vi "vision_webcam_V6.vi"() -> ()   [LabVIEW 2017]
uses:
  <vilib>/userdefined/High Color/IMAQdx.ctl
  <vilib>/vision/Image Controls.llb/IMAQ Image.ctl
  <vilib>/vision/Avi.llb/IMAQ AVI2 Codec Path.ctl
  Globals/Global - All RT Loop Stop.vi
  <vilib>/vision/driver/NI_Vision_Acquisition_Software.lvlib
panel:
  out "error out":errorcluster
  in  "y":bool
  out "AVI Path":path
  out "concatenated string 2":string
  in  "Boolean":bool
  out "Codec Names":string[](array[string])
  out "Webcam":T1(plugin-control)
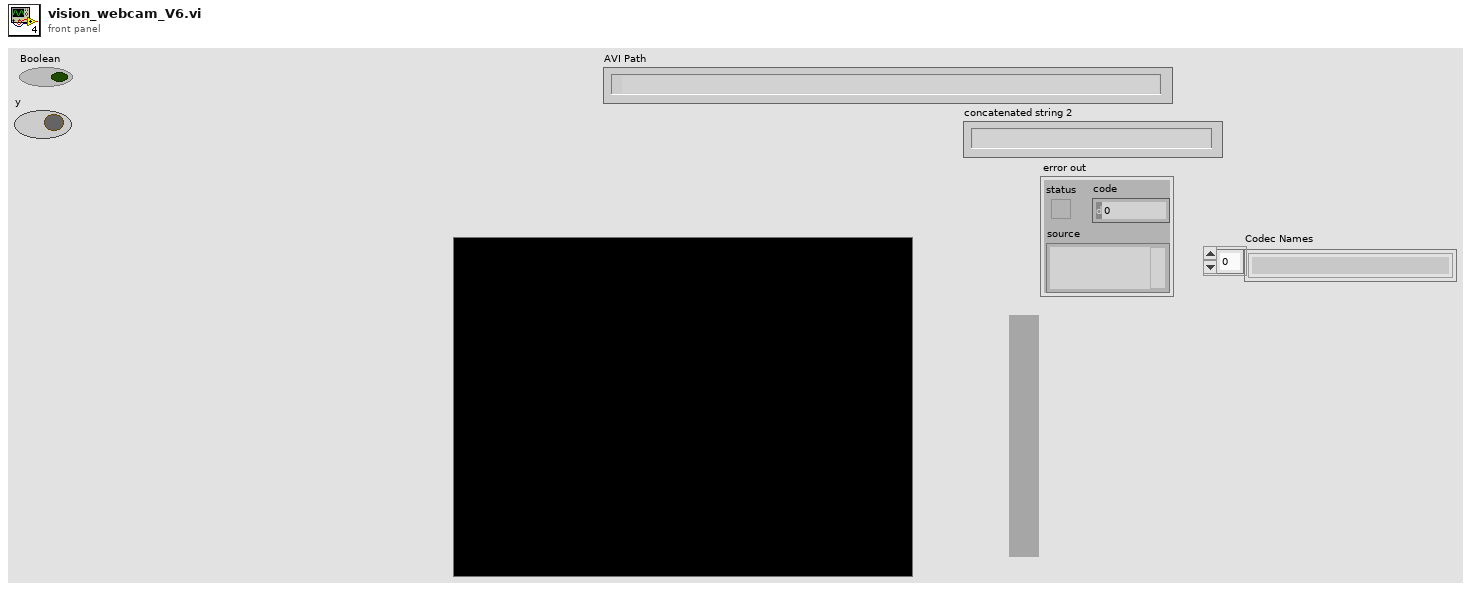
[diagram p1: front panel]
types:
  T1 = typedef "IMAQ Image.ctl" = refnum<image>
  T2 = typedef "IMAQdx.ctl" = refnum<k21>
  T3 = typedef "Image Type" = u32
  T4 = typedef "IMAQ AVI2 Refnum.ctl" = refnum<k20>
  T5 = typedef "IMAQ AVI2 Codec Path.ctl" = u32
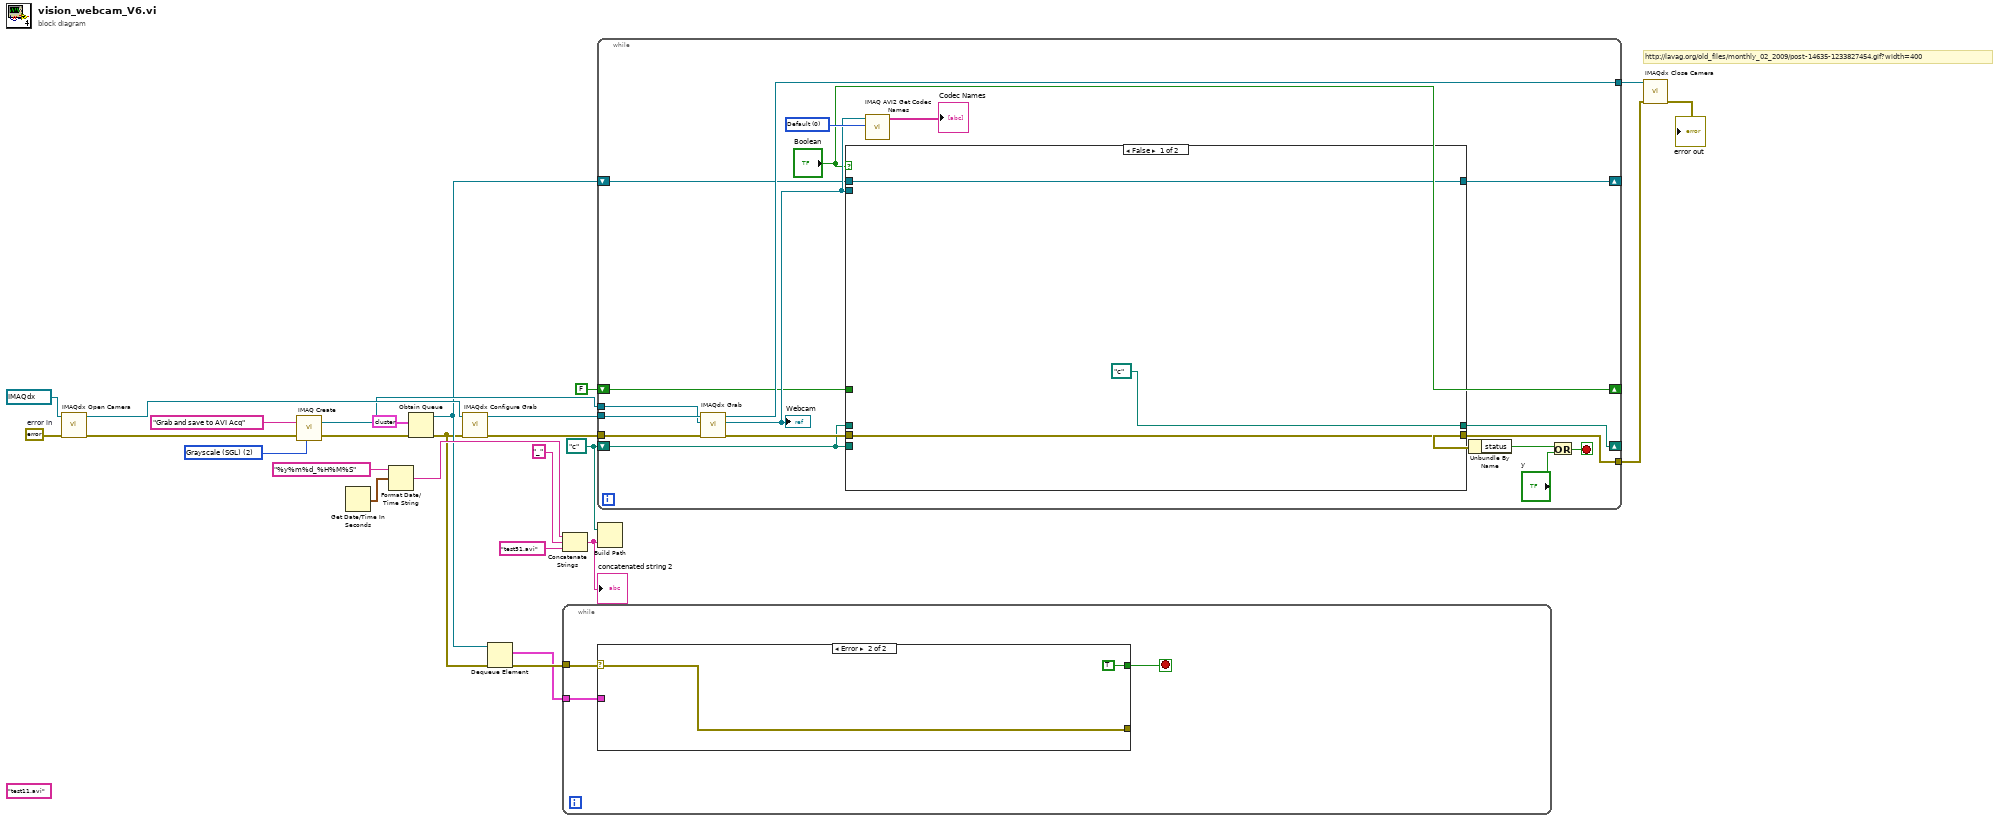
[diagram p0: block diagram]
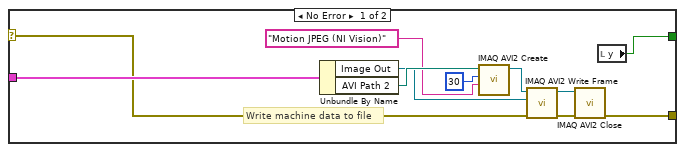
[diagram p2: hidden frame]
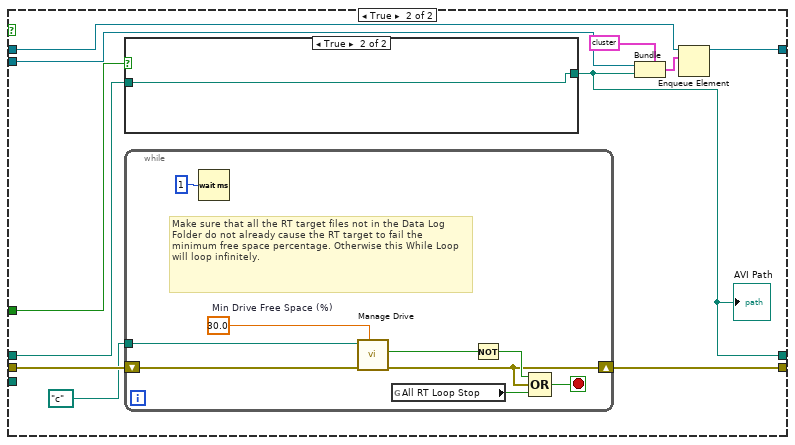
[diagram p3: hidden frame]
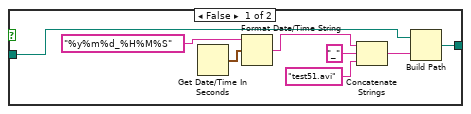
[diagram p4: hidden frame]
diagram:
  (unwired) "test11.avi" ("name or relative path")
  w11 = path "c:/" ("AVI Path")
  w21 = T3 2 items=["Grayscale (U8)", "Grayscale (I16)", "Grayscale (SGL)", "Complex (CSG)", "RGB (U32)", "HSL (U32)", "RGB (U64)", "Grayscale (U16)"] ("Image Type")
  w23 = errorcluster {"status"=FALSE, "code"=0, "source"=""}  # error in
  # "http://lavag.org/old_files/monthly_02_2009/post-14635-1233827454.gif?width=400"
  n1 = call <vilib>:"IMAQdx Open Camera.vi"("error in"=w23, "Session In"=T2 "cam0") -> ("error out"=w20:errorcluster, "Session Out"=w25:T2)  [unwired: 8 in]
  n2 = call "IMAQ Create"("Image Name"="Grab and save to AVI Acq", "Image Type"=w21, "error in (no error)"=w20) -> ("New Image"=w17:T1, "error out"=w4:errorcluster)  [unwired: 2 in]
  n3 = Get Date/Time In Seconds() -> (seconds since 1Jan1904=w15:timestamp)
  n4 = Format Date/Time String(time format string (%c)="%y%m%d_%H%M%S", seconds (now)=w15) -> (date/time string=w14:string)  [unwired: 1 out]
  n5 = Obtain Queue(element data type=cluster{"Image Out":T1, "AVI Path 2":path} {"Image Out"=refnum, "AVI Path 2"=path ""}, error in (no error)=w4) -> (queue out=w5:refnum<queue>, error out=w3:errorcluster)  [unwired: 3 in, 1 out]
  n6 = call <vilib>:"IMAQdx Configure Grab.vi"("error in"=w3, "Session In"=w25) -> ("error out"=w18:errorcluster, "Session Out"=w19:T2)  [unwired: 8 in]
  n7 = Dequeue Element(queue=w5, error in (no error)=w3) -> (element=w6:cluster{"Image Out":T1, "AVI Path 2":path}, error out=w7:errorcluster)  [unwired: 1 in, 2 out]
  n8 = Concatenate Strings(w14, "_" ("string"), "test51.avi" ("name or relative path")) -> (w10:string)
  "concatenated string 2" <- w10
  n9 = while {
    tunnel: w7 -> [w29]
    tunnel: w6 -> [w28]
    stop <- w27 stop-if-true
    n10 = case shown="Error" w29 {
      selector: w29 -> [w34 w42]
      tunnel: [w31 w42] -> _
      tunnel: w28 -> [w40 _]
      tunnel: [w30 TRUE] -> w27
      frame No Error {
        # "Write machine data to file"
        n11 = Unbundle By Name(w40) -> ("Image Out"=w35:T1, "AVI Path 2"=w39:path)
        n12 = call "IMAQ AVI2 Create"("Codec"="Motion JPEG (NI Vision)", "Frames Per Second"=u32 30, "AVI Path"=w39) -> ("AVI Refnum"=w36:T4)  [unwired: 7 in, 1 out]
        n13 = call "IMAQ AVI2 Write Frame"("error in (no error)"=w34, "Image"=w35, "AVI Refnum"=w36) -> ("error out"=w32:errorcluster, "AVI Refnum (duplicate)"=w33:T4)  [unwired: 6 in, 1 out]
        n14 = call "IMAQ AVI2 Close"("error in (no error)"=w32, "AVI Refnum"=w33) -> ("error out"=w31:errorcluster)  [unwired: 9 in]
        n15 = local read "y"() -> (w30:bool)
      }
      frame Error {
      }
    }
  }
  n16 = while {
    tunnel: w18 -> [w60]
    tunnel: w19 -> [w59]
    tunnel: w17 -> [w58]
    tunnel: [w50] -> w2
    tunnel: [w57] -> w26
    shift-right: [w48] -> _
    shift-left: w5 -> [w49]
    shift-right: ["Boolean"] -> _
    shift-left: FALSE ("G1 trigger") -> [w47]
    shift-right: [w44] -> _
    shift-left: w11 -> [w45]
    stop <- w55 stop-if-true
    w54 = T5 0 items=["Default", "System", "Built in Vision"] ("Codec Source")
    n17 = call <vilib>:"IMAQdx Grab.vi"("error in"=w60, "Image In"=w58, "Session In"=w59) -> ("error out"=w51:errorcluster, "Image Out"=w52:T1, "Session Out"=w57:T2)  [unwired: 5 in, 1 out]
    "Webcam" <- w52
    n18 = case shown="False" "Boolean" {
      tunnel: w52 -> [_ w67]
      tunnel: w51 -> [w63 w65]
      tunnel: [w63 w74] -> w50
      tunnel: w45 -> [_ _]
      tunnel: w49 -> [w62 w73]
      tunnel: [w62 w72] -> w48
      tunnel: w47 -> [_ w71]
      tunnel: w45 -> [_ w70]
      tunnel: [path "c:/" ("AVI Path") w68] -> w44
      frame False {
      }
      frame True {
        n19 = case shown="True" w71 {
          tunnel: w70 -> [w76 w83]
          tunnel: [w75 w83] -> w68
          frame False {
            n20 = Get Date/Time In Seconds() -> (seconds since 1Jan1904=w78:timestamp)
            n21 = Format Date/Time String(time format string (%c)="%y%m%d_%H%M%S", seconds (now)=w78) -> (date/time string=w79:string)  [unwired: 1 out]
            n22 = Concatenate Strings(w79, "_" ("string"), "test51.avi" ("name or relative path")) -> (w82:string)
            n23 = Build Path(base path=w76, name or relative path=w82) -> (appended path=w75:path)
          }
          frame True {
          }
        }
        "AVI Path" <- w68
        n24 = while {
          shift-right: [w87] -> w74
          shift-left: w65 -> [w88]
          tunnel: path "c:/" ("AVI Path") -> [w85]
          stop <- w92 stop-if-true
          w86 = 30.0  # Min Drive Free Space (%)
          # "Make sure that all the RT target files not in the Data Log Folder do not already cause the RT target to fail the minimum free space percentage. Otherwise this While Loop will loop infinitely."
          n25 = Wait (ms)(milliseconds to wait=u32 1) -> ()  [unwired: 1 out]
          n26 = call "Manage Drive.vi"("Min Drive Free Space (%)"=w86, "error in"=w88, "Data Folder"=w85) -> ("error out"=w87:errorcluster, "Drive Space Below Limit"=w84:bool)  [unwired: 6 in, 1 out]
          n27 = global read "Global - All RT Loop Stop.vi" "All RT Loop Stop"() -> (w89:bool)
          n28 = Not(x=w84) -> (.not. x?=w91:bool)
          n29 = Compound Arithmetic op=OR(w91, w87, w89) -> (w92:bool)
        }
        n30 = Bundle(cluster=cluster{"Image Out":T1, "AVI Path 2":path} {"Image Out"=refnum, "AVI Path 2"=path ""}, "Image Out"=w67, "AVI Path 2"=w68) -> (w66:cluster{"Image Out":T1, "AVI Path 2":path})
        n31 = Enqueue Element(queue=w73, element=w66) -> (queue out=w72:refnum<queue>)  [unwired: 2 in, 2 out]
      }
    }
    n32 = call "IMAQ AVI2 Get Codec Names"("Codec Source"=w54, "Image"=w52) -> ("Codec Names"=→"Codec Names":string[])  [unwired: 8 in, 1 out]
    n33 = Unbundle By Name(w50) -> ("status"=w56:bool)
    n34 = Or(x=w56, y="y") -> (x .or. y?=w55:bool)
  }
  n35 = Build Path(base path=w11, name or relative path=w10) -> ()  [unwired: 1 out]
  n36 = call <vilib>:"IMAQdx Close Camera.vi"("error in"=w2, "Session In"=w26) -> ("error out"=→"error out":errorcluster)  [unwired: 9 in]
